vi "Timestamp Blocking Read.vi"(8 "error in (no error)":errorcluster, 10 "RX Time":i64, 11 "CIFCorePlugin in":refnum<class "CIFCorePlugin.lvclass">) -> (0 "error out":errorcluster, 3 "CIFCorePlugin out":refnum<class "CIFCorePlugin.lvclass">)   [LabVIEW 2021, in "CIFCorePlugin.lvclass"]
doc: "This can be used to provide timestamps for plugins that are configured to \"Skip Sleep\" and use a blocking read (FIFO or driver call) to control timing."
uses:
  CIFCorePlugin.lvclass
  CIFCorePlugin.lvclass/CIFCorePlugin.ctl
  <vilib>/CIF Foundation/CIF Utilities/Time/System Time/Get System Time.vi
  <vilib>/CIF Foundation/CIF Utilities/Time/System Time/LabVIEW Time to TAI Time.vi
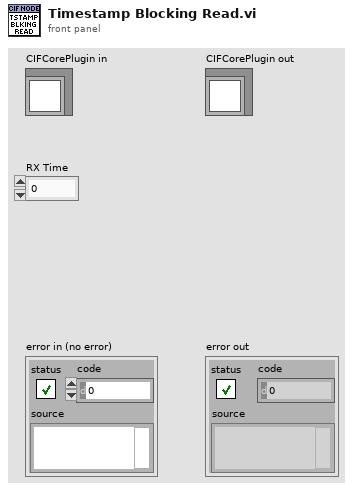
[diagram p1: front panel]
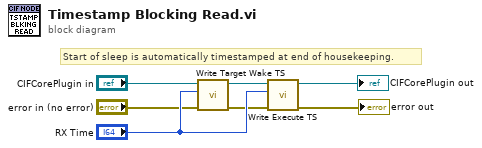
[diagram p0: block diagram]
diagram:
  # "Start of sleep is automatically timestamped at end of housekeeping."
  n1 = call "Write Target Wake TS.vi"("error in (no error)"="error in (no error)", "Target Wake"="RX Time", "CIFCorePlugin in"="CIFCorePlugin in") -> ("error out"=w2:errorcluster, "CIFCorePlugin out"=w1:refnum<class "CIFCorePlugin.lvclass">)  [unwired: 7 in]
  n2 = call "Write Execute TS.vi"("error in (no error)"=w2, "Execute"="RX Time", "CIFCorePlugin in"=w1) -> ("error out"=→"error out":errorcluster, "CIFCorePlugin out"=→"CIFCorePlugin out":refnum<class "CIFCorePlugin.lvclass">)  [unwired: 7 in]
